vi "Autosize Table Columns.vi"(4 "error in (no error)":errorcluster, 6 "Resize Table?":bool, 7 "Table Ref":refnum<vi>) -> (0 "error out":errorcluster)   [LabVIEW 2014]
doc: "This VI resizes each column of the table specified by Table Ref based on the widest entry of the column. Additionally, if Resize Table? is TRUE, the VI will set the table width based on the number of populated columns."
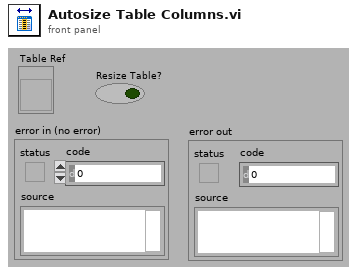
[diagram p1: front panel]
types:
  T1 = enum16{"User-specified Font", "Application Font", "System Font", "Dialog Font"}
  T2 = cluster{"Font Name:":string, "Size":i16, "Strikeout?":bool, "Italic?":bool, "Underline?":bool, "Outline?":bool, "Shadow?":bool, "Bold?":bool}
  T3 = cluster{"left":i16, "top":i16, "right":i16, "bottom":i16}
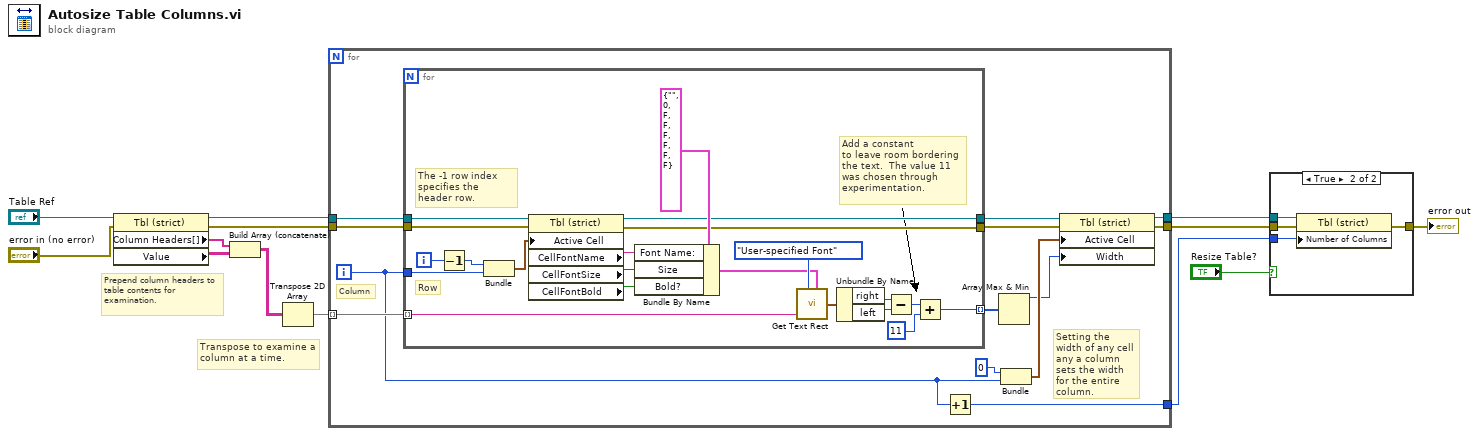
[diagram p0: block diagram]
diagram:
  # "Transpose to examine a column at a time."
  # "Prepend column headers to table contents for examination."
  n1 = property class="Tbl (strict)"(reference="Table Ref", error in="error in (no error)") -> (reference out=w13:refnum<vi>, error out=w9:errorcluster, "Column Headers[]"=w12:string[], "Value"=w8:string[][])
  n2 = Build Array (concatenate)(w12, w8) -> (w11:string[][])
  n3 = Transpose 2D Array(2D array=w11) -> (transposed array=w10:string[][])
  n4 = for {
    tunnel: w10 -> [w26] mode=indexing
    tunnel: w13 -> [w25]
    tunnel: w9 -> [w23]
    tunnel: [w17] -> w3
    tunnel: [w16] -> w4
    tunnel: [w14] -> w2
    i -> [w15]
    # "Setting the width of any cell any a column sets the width for the entire column."
    # "Column"
    n5 = for {
      tunnel: w26 -> [w39] mode=indexing
      tunnel: w25 -> [w47]
      tunnel: w15 -> [w46]
      tunnel: [w28] -> w24 mode=indexing
      tunnel: w23 -> [w33]
      tunnel: [w32] -> w21
      tunnel: [w31] -> w22
      i -> [w35]
      # "The -1 row index specifies the header row."
      # "Add a constant\nto leave room bordering the text.  The value 11 was chosen through experimentation."
      # "Row"
      n6 = Decrement(x=w35) -> (x-1=w34:i32)
      n7 = Bundle(w34, w46) -> (w45:cluster{i32, i32})  [unwired: 1 in]
      n8 = property class="Tbl (strict)"(reference=w47, error in=w33, "Active Cell"=w45) -> (reference out=w31:refnum<vi>, error out=w32:errorcluster, "CellFontName"=w43:string, "CellFontSize"=w29:u32, "CellFontBold"=w42:bool)
      n9 = Bundle By Name(cluster=T2 {"Font Name:"="", "Size"=0, "Strikeout?"=FALSE, "Italic?"=FALSE, "Underline?"=FALSE, "Outline?"=FALSE, "Shadow?"=FALSE, "Bold?"=FALSE} ("[user-specified font]"), "Font Name:"=w43, "Size"=w29, "Bold?"=w42) -> (w40:T2)
      n10 = call <vilib>:"Get Text Rect.vi"("desired font(Application)"=T1."User-specified Font", "text"=w39, "[user-specified font]"=w40) -> ("rect"=w38:T3)  [unwired: 6 in]
      n11 = Unbundle By Name(w38) -> ("right"=w37:i16, "left"=w36:i16)
      n12 = Subtract(x=w37, y=w36) -> (x-y=w30:i16)
      n13 = Add(x=w30, y=i16 11) -> (x+y=w28:i16)
    }
    n14 = Increment(x=w15) -> (x+1=w14:i32)
    n15 = Array Max & Min(array=w24) -> (max value=w18:i16)  [unwired: 3 out]
    n16 = Bundle(0, w15) -> (w19:cluster{i32, i32})  [unwired: 1 in]
    n17 = property class="Tbl (strict)"(reference=w22, error in=w21, "Active Cell"=w19, "Width"=w18) -> (reference out=w16:refnum<vi>, error out=w17:errorcluster)
  }
  n18 = case shown="True" "Resize Table?" {
    tunnel: w4 -> [_ w52]
    tunnel: w3 -> [w48 w51]
    tunnel: w2 -> [_ w50]
    tunnel: [w48 w49] -> w1
    frame False {
    }
    frame True {
      n19 = property class="Tbl (strict)"(reference=w52, error in=w51, "Number of Columns"=w50) -> (error out=w49:errorcluster)  [unwired: 1 out]
    }
  }
  "error out" <- w1
